vi "FlatSequence.vi"() -> ()   [LabVIEW 2017]
panel:
  out "number (0 to 1)":dbl
  in  "stop":bool
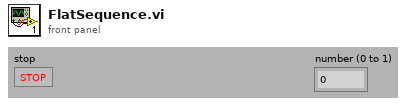
[diagram p1: front panel]
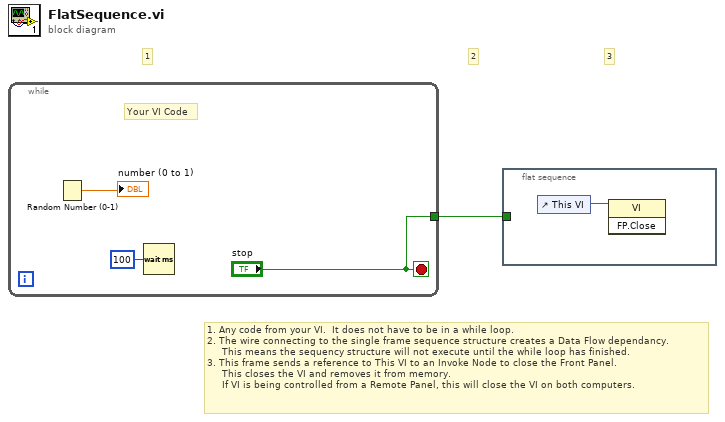
[diagram p0: block diagram]
diagram:
  # "1. Any code from your VI.  It does not have to be in a while loop.\n2. The wire connecting to the single frame sequence structure creates a Data Flow dependancy.\n     This means the sequency structure will not execute until the while loop has finished.\n3. This frame sends a reference to This VI to an Invoke Node to close the Front Panel.\n     This closes the VI and removes it from memory.\n     If VI is being controlled from a Remote Panel, this will close the VI on both computers."
  # "3"
  # "2"
  # "1"
  n1 = while {
    tunnel: ["stop"] -> w1
    stop <- "stop" stop-if-true
    # "Your VI Code"
    n2 = Random Number (0-1)() -> (number: 0 to 1=→"number (0 to 1)":dbl)
    n3 = Wait (ms)(milliseconds to wait=u32 100) -> ()  [unwired: 1 out]
  }
  n4 = flat-sequence {
    tunnel: w1 -> [_]
    frame #0 {
      n5 = control-ref of="This VI"() -> (w5:refnum<vi>)
      n6 = invoke class="VI" method="FP.Close"(reference=w5) -> ()  [unwired: 2 in, 3 out]
    }
  }
